vi "get_path_exe.vi"(8 "error in (no error)":errorcluster) -> (0 "error out":errorcluster, 3 "exe":path)   [LabVIEW 2015, in "lv-bin-7zip.lvlib"]
uses:
  lv-bin-7zip.lvlib
  public/_controls/error.ctl
  <userlib>/antonio-alexander/lv-bin/lv-bin/public/api/v1/v1.lvlib
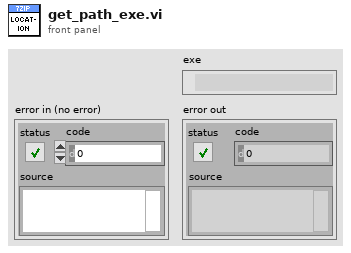
[diagram p1: front panel]
types:
  T1 = typedef "lv-bin-7zip.lvlib/error.ctl" = enum16{"null", "exe_x86_missing", "exe_x64_missing", "7za_x86_missing", "7za_x64_missing", "7zxa_x86_missing", "7zxa_x64_missing", "7zS.sfx_missing"}
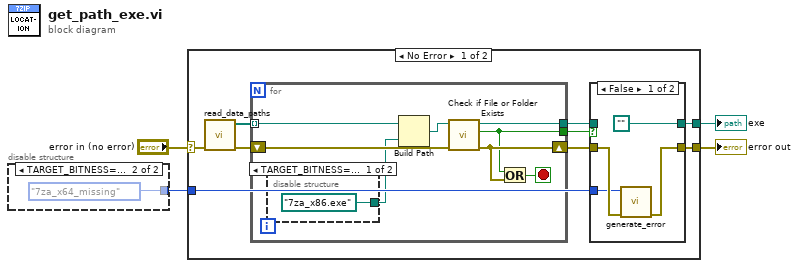
[diagram p0: block diagram]
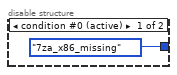
[diagram p2: hidden frame]
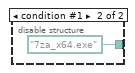
[diagram p3: hidden frame]
diagram:
  n1 = disable-structure shown="TARGET_BITNESS==64" {
    disable-tunnel: [error."7za_x86_missing" ("error") error."7za_x64_missing" ("error")] -> w1
    frame condition #0 (active) {
    }
    frame condition #1 {
    }
  }
  n2 = case shown="No Error" "error in (no error)" {
    selector: "error in (no error)" -> [w15 w32]
    tunnel: [w8 w32] -> w2
    tunnel: [w10 _] -> w4
    tunnel: w1 -> [w7 _]
    frame No Error {
      n3 = call <userlib>:"read_data_paths.vi"("error in (no error)"=w15) -> ("error out"=w14:errorcluster, "path [] out"=w13:path[])  [unwired: 9 in]
      n4 = for {
        tunnel: w13 -> [w21] mode=indexing
        shift-right: [w20] -> w9
        shift-left: w14 -> [w23]
        tunnel: [w22] -> w12
        tunnel: [w18] -> w11
        stop <- w19 stop-if-true
        n5 = disable-structure shown="TARGET_BITNESS==32, Default" {
          disable-tunnel: [path "7za_x86.exe" ("Application Directory") path "7za_x64.exe" ("Application Directory")] -> w16
          frame condition #0 (active) {
          }
          frame condition #1 {
          }
        }
        n6 = Build Path(base path=w21, name or relative path=w16) -> (appended path=w17:path)
        n7 = call <vilib>:"Check if File or Folder Exists.vi"("error in (no error)"=w23, "path"=w17) -> ("error out"=w20:errorcluster, "file or folder exists?"=w18:bool, "dup path"=w22:path)  [unwired: 7 in]
        n8 = Or(x=w18, y=w20) -> (x .or. y?=w19:bool)
      }
      n9 = case shown="False" w11 {
        tunnel: w12 -> [_ w31]
        tunnel: [path "" w31] -> w10
        tunnel: w9 -> [w29 w30]
        tunnel: [w28 w30] -> w8
        tunnel: w7 -> [w26 _]
        frame False {
          n10 = call "generate_error.vi"("error in (no error)"=w29, "error"=w26) -> ("error out"=w28:errorcluster)  [unwired: 9 in]
        }
        frame True {
        }
      }
    }
    frame Error {
    }
  }
  "error out" <- w2
  "exe" <- w4
